vi "Autonomous Independent.vi"() -> ()   [LabVIEW 2012]
doc: "This VI is called when autonomous begins, and will automatically be terminated when autonomous ends. You can carry out timed or sensor driven robot movement independently without needing to return to the caller."
uses:
  <vilib>/Rock Robotics/WPI/RobotDrive/WPI_RobotDriveArcadeDrive_Standard(NoSaturation).vi
  Robot Global Data.vi
  <vilib>/Rock Robotics/WPI/Solenoid/WPI_SolenoidSetEnum.vi
  <vilib>/Rock Robotics/WPI/Solenoid/WPI_SolenoidValue.ctl
  <vilib>/Rock Robotics/WPI/CAN/Jaguar/SubVIs/WPI_CANJaguar_ControlMode.ctl
  <vilib>/Rock Robotics/WPI/CAN/Jaguar/SubVIs/WPI_CANJaguar_PositionReference.ctl
panel:
  out "Current Movement, for debugging":T1 {"Y Joystick Value" scale=1.0..-1.0; "X Joystick Value" scale=-1.0..1.0}
  in  "Array of robot movements":T2(array[cluster]) {"Y Joystick Value" scale=1.0..-1.0; "X Joystick Value" scale=-1.0..1.0}
  # "Be sure to right-click and choose Data Operations>>Make Current Value default if you want to save the array values with the VI"
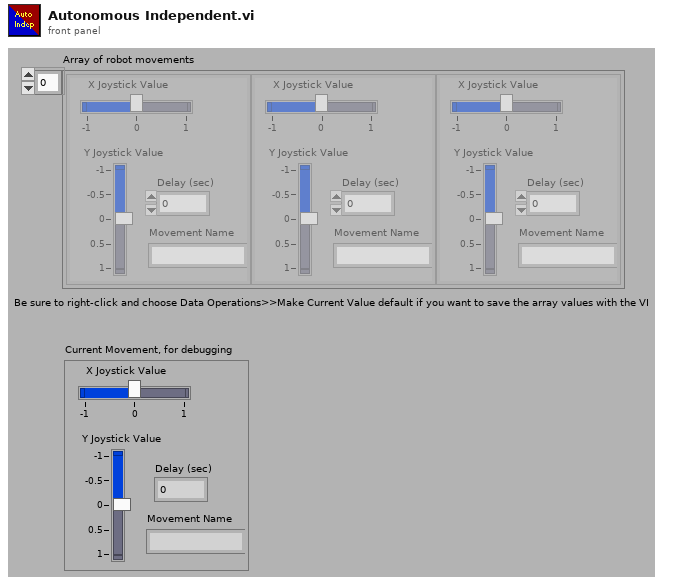
[diagram p1: front panel]
types:
  T1 = cluster{"X Joystick Value":dbl, "Y Joystick Value":dbl, "Delay (sec)":dbl, "Movement Name":string}
  T2 = cluster{"X Joystick Value":dbl, "Y Joystick Value":dbl, "Delay (sec)":dbl, "Movement Name":string}[]
  T3 = typedef "WPI_JoystickDevRef.ctl" = cluster{"Device":T4}
  T4 = typedef "WPI_JoystickDeviceEnum.ctl" = enum16{"USB 1", "USB 2", "USB 3", "USB 4", "Kinect 1", "Kinect 2"}
  T5 = cluster{"axis 1 (x)":dbl, "axis 2 (y)":dbl, "axis 3 (throttle)":dbl, "axis 4":dbl, "axis 5":dbl, "axis 6":dbl}
  T6 = typedef "WPI_SolenoidValue.ctl" = enum16{"Off", "On", "Forward", "Reverse"}
  T7 = typedef "WPI_CANJaguar_ControlMode.ctl" = enum8{"Percent VBus", "Current", "Speed", "Position", "Voltage"}
  T8 = typedef "WPI_SolenoidDevRef.ctl" = cluster{"DevStatus":errorcluster, "Solenoid Module":T9, "Forward Solenoid Channel":T10, "Reverse Solenoid Channel":T10}
  T9 = typedef "FPGA_TypedefSolenoidModule.ctl" = enum16{"Solenoid Module 1", "Solenoid Module 2"}
  T10 = typedef "WPI_SolenoidChannel.ctl" = enum8{"Solenoid 1", "Solenoid 2", "Solenoid 3", "Solenoid 4", "Solenoid 5", "Solenoid 6", "Solenoid 7", "Solenoid 8", "Invalid"}
  T11 = typedef "WPI_MotorControlDeviceRef.ctl" = cluster{"DeviceStatus":errorcluster, "Type":enum16{"PWM", "CAN"}, "PWM":cluster{"Digital Module":T12, "PWM Channel":T13, "DeadBand":T14}, "CAN":cluster{"Device Number":u8, "Control Mode":T7, "Semaphore":T15, "Max Vout":dbl}, "Invert":bool, "TransformRef":T16, "InvTransformRef":T16}
  T12 = typedef "FPGA_TypedefDigitalModule.ctl" = enum16{"Digital Module 1", "Digital Module 2"}
  T13 = typedef "FPGA_DIOPWMChannel.ctl" = enum8{"PWM 1", "PWM 2", "PWM 3", "PWM 4", "PWM 5", "PWM 6", "PWM 7", "PWM 8", "PWM 9", "PWM 10", "Invalid"}
  T14 = typedef "WPI_PWMDeadband.ctl" = cluster{"Name":string, "maxPositivePwm":i32, "minPositivePwm":i32, "centerPwm":i32, "maxNegativePwm":i32, "minNegativePwm":i32, "angularRange":u16}
  T15 = typedef "Semaphore RefNum" = refnum<k1>
  T16 = typedef "WPI_PWMTransform_ConPane.ctl" = refnum<vi>
  T17 = typedef "WPI_CANJaguar_PositionReference.ctl" = u8
  T18 = typedef "WPI_RobotDriveDevRef.ctl" = cluster{"DevStatus":errorcluster, "Motors[]":T11[], "Square Inputs":bool, "Max Output":dbl, "Isochronous":bool}
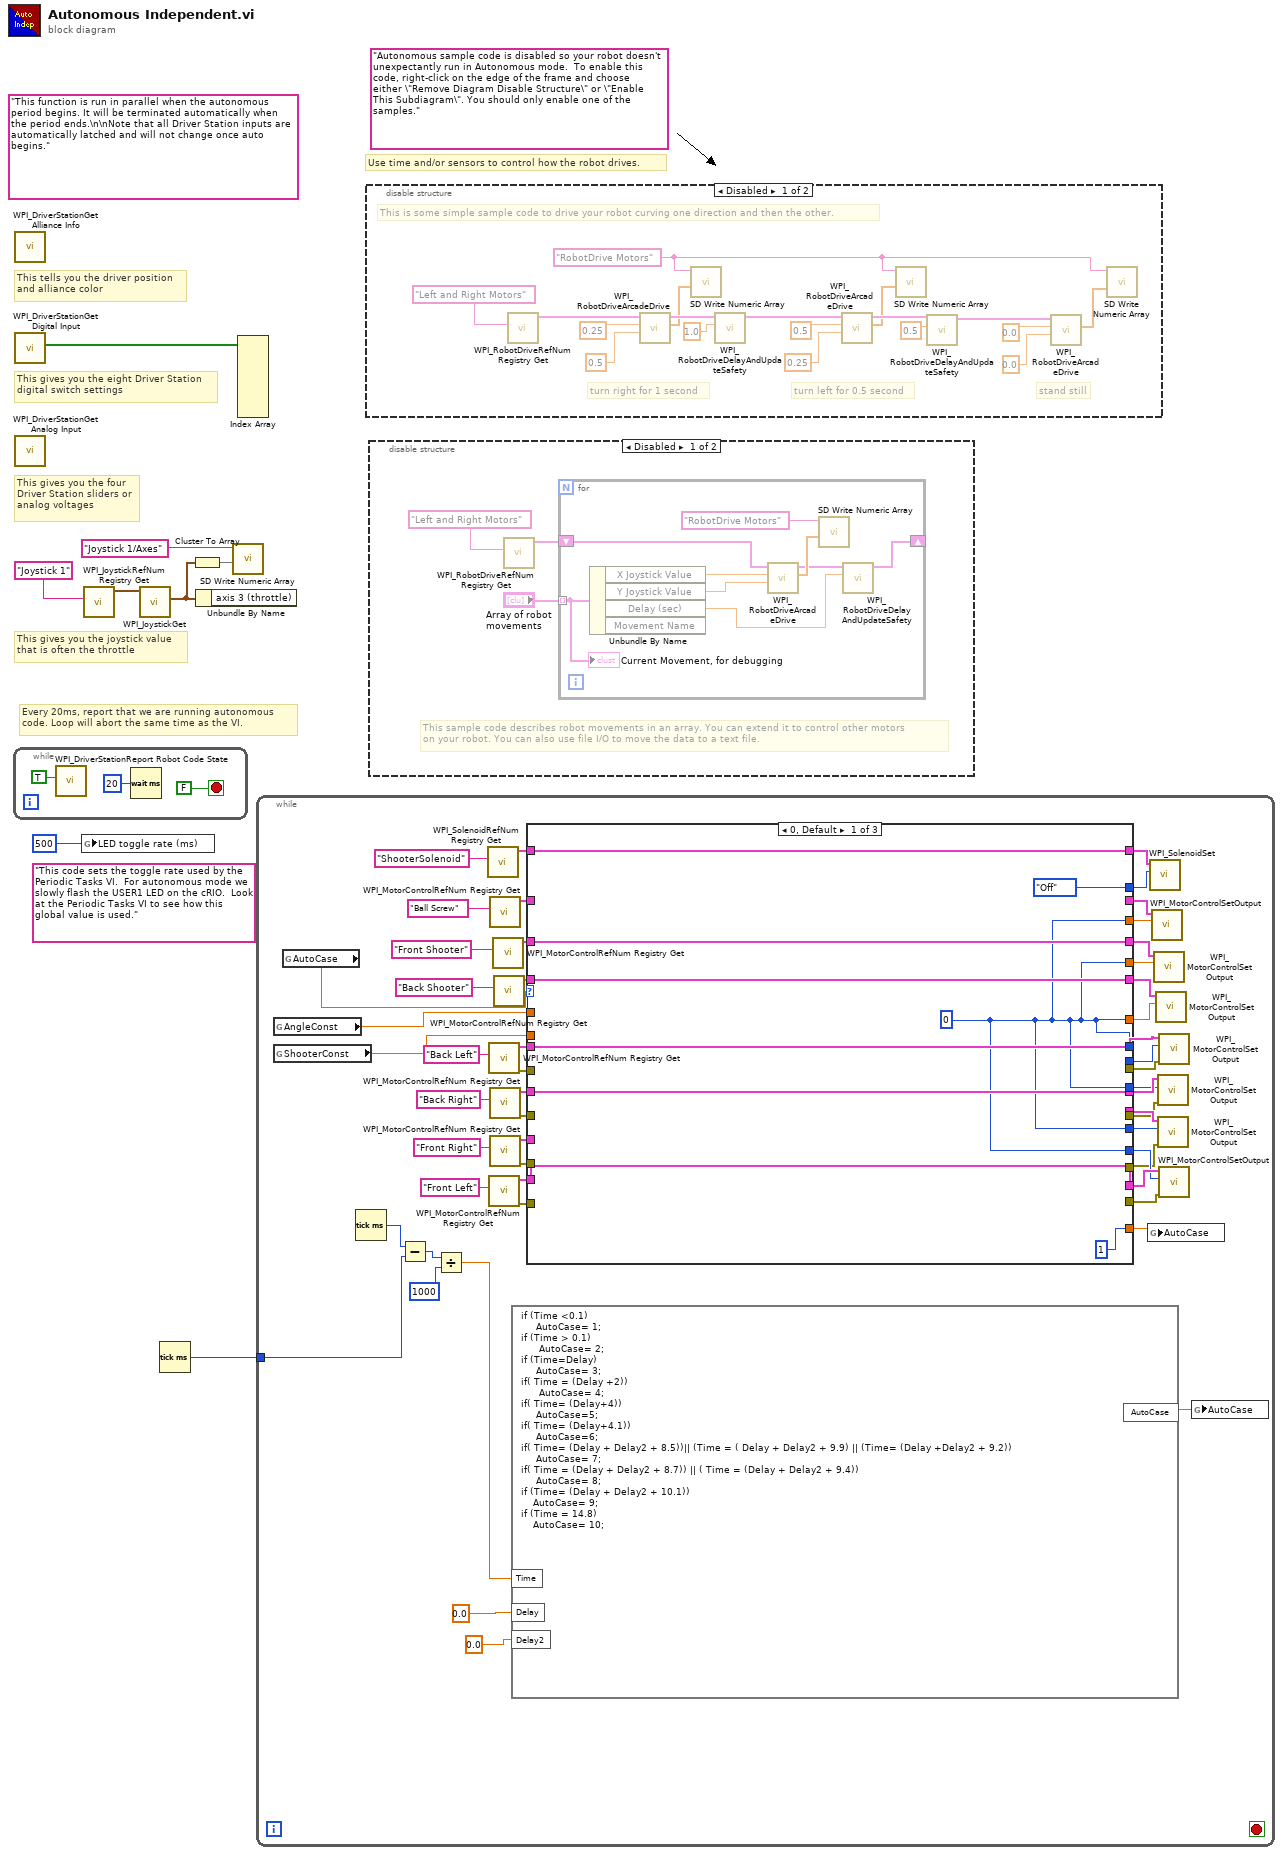
[diagram p0: block diagram]
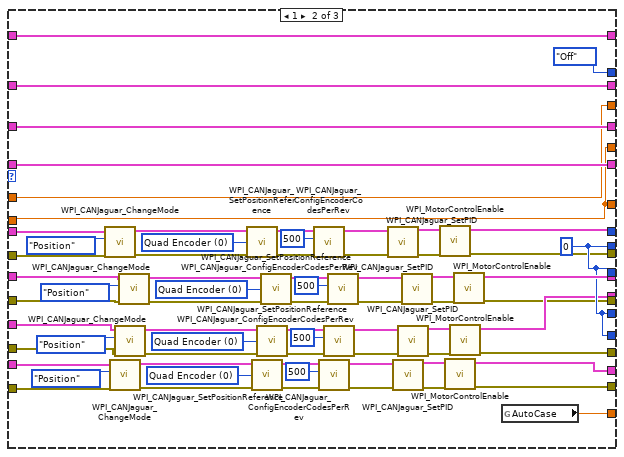
[diagram p2: hidden frame]
diagram:
  (unwired) "This code sets the toggle rate used by the Periodic Tasks VI.  For autonomous mode we slowly flash the USER1 LED on the cRIO.  Look at the Periodic Tasks VI to see how this global value is used."
  (unwired) "Autonomous sample code is disabled so your robot doesn't unexpectantly run in Autonomous mode.  To enable this code, right-click on the edge of the frame and choose either \"Remove Diagram Disable Structure\" or \"Enable This Subdiagram\". You should only enable one of the samples."
  (unwired) "This function is run in parallel when the autonomous period begins. It will be terminated automatically when the period ends.\n\nNote that all Driver Station inputs are automatically latched and will not change once auto begins."
  # "Every 20ms, report that we are running autonomous\ncode. Loop will abort the same time as the VI."
  # "This gives you the joystick value\nthat is often the throttle"
  # "Use time and/or sensors to control how the robot drives."
  # "This tells you the driver position\nand alliance color"
  # "This gives you the eight Driver Station\ndigital switch settings"
  # "This gives you the four\nDriver Station sliders or\nanalog voltages"
  n1 = while {
    stop <- FALSE stop-if-true
    n2 = call <vilib>:"WPI_DriverStationReport Robot Code State.vi"("Autonomous"=TRUE) -> ()  [unwired: 10 in, 1 out]
    n3 = Wait (ms)(milliseconds to wait=u32 20) -> ()  [unwired: 1 out]
  }
  n4 = call <vilib>:"WPI_DriverStationGet Alliance Info.vi"() -> ()  [unwired: 12 out]
  n5 = call <vilib>:"WPI_DriverStationGet Digital Input.vi"() -> ("Driver Station Digital Input (1-8)"=w8:bool[])  [unwired: 11 out]
  n6 = call <vilib>:"WPI_DriverStationGet Analog Input.vi"() -> ()  [unwired: 12 out]
  n7 = global write "Robot Global Data.vi" "LED toggle rate (ms)"(u32 500 ("LED ms toggle rate")) -> ()
  n8 = call <vilib>:"WPI_JoystickRefNum Registry Get.vi"("refnum name"="Joystick 1") -> ("JoystickDevRef"=w6:T3)  [unwired: 1 in, 9 out]
  n9 = call <vilib>:"WPI_JoystickGet.vi"("JoystickDevRef"=w6) -> ("Axes"=w3:T5)  [unwired: 1 in, 5 out]
  n10 = Tick Count (ms)() -> (millisecond timer value=w1:u32)
  n11 = Cluster To Array(cluster=w3) -> (array=w4:dbl[])
  n12 = Unbundle By Name(w3) -> ()  [unwired: 1 out]
  n13 = call <vilib>:"SD Write Numeric Array.vi"("Numeric Array"=w4, "Name"="Joystick 1/Axes") -> ()  [unwired: 8 in, 2 out]
  n14 = Index Array(array=w8) -> ()  [unwired: 8 in, 8 out]
  n15 = while {
    tunnel: w1 -> [w52]
    stop <- _ stop-if-true
    n16 = global read "Robot Global Data.vi" "AngleConst"() -> (w13:dbl)
    n17 = global read "Robot Global Data.vi" "ShooterConst"() -> (w12:dbl)
    n18 = global read "Robot Global Data.vi" "AutoCase"() -> (w54:dbl)
    n19 = Tick Count (ms)() -> (millisecond timer value=w53:u32)
    n20 = Subtract(x=w53, y=w52) -> (x-y=w51:u32)
    n21 = Divide(x=w51, y=u32 1000) -> (x/y=w49:dbl)
    n22 = call <vilib>:"WPI_SolenoidRefNum Registry Get.vi"("refnum name"="ShooterSolenoid") -> ("SolenoidDevRef"=w55:T8)  [unwired: 9 in, 1 out]
    n23 = call <vilib>:"WPI_MotorControlRefNum Registry Get.vi"("refnum name"="Back Left") -> ("error out"=w25:errorcluster, "MotorControlDevRef"=w37:T11)  [unwired: 9 in]
    n24 = call <vilib>:"WPI_MotorControlRefNum Registry Get.vi"("refnum name"="Front Left") -> ("error out"=w15:errorcluster, "MotorControlDevRef"=w33:T11)  [unwired: 9 in]
    n25 = call <vilib>:"WPI_MotorControlRefNum Registry Get.vi"("refnum name"="Ball Screw") -> ("MotorControlDevRef"=w26:T11)  [unwired: 9 in, 1 out]
    n26 = call <vilib>:"WPI_MotorControlRefNum Registry Get.vi"("refnum name"="Back Right") -> ("error out"=w23:errorcluster, "MotorControlDevRef"=w35:T11)  [unwired: 9 in]
    n27 = call <vilib>:"WPI_MotorControlRefNum Registry Get.vi"("refnum name"="Front Right") -> ("error out"=w19:errorcluster, "MotorControlDevRef"=w21:T11)  [unwired: 9 in]
    n28 = call <vilib>:"WPI_MotorControlRefNum Registry Get.vi"("refnum name"="Front Shooter") -> ("MotorControlDevRef"=w41:T11)  [unwired: 9 in, 1 out]
    n29 = call <vilib>:"WPI_MotorControlRefNum Registry Get.vi"("refnum name"="Back Shooter") -> ("MotorControlDevRef"=w39:T11)  [unwired: 9 in, 1 out]
    n30 = formula code="if (Time <0.1)\n     AutoCase= 1;\nif (Time > 0.1)\n      AutoCase= 2;\nif (Time=Delay)\n     AutoCase= 3;\nif( Time = (Delay +2))\n      AutoCase= 4;\nif( Time= (Delay+4))\n     AutoCase=5;\nif( Time= (Delay+4.1))\n     AutoCase=6;\nif( Time= (Delay + Delay2 + 8.5))|| (Time = ( Delay + Delay2 + 9.9) || (Time= (Delay +Delay2 + 9.2))\n     AutoCase= 7;\nif( Time = (Delay + Delay2 + 8.7)) || ( Time = (Delay + Delay2 + 9.4))\n     AutoCase= 8;\nif (Time= (Delay + Delay2 + 10.1))\n    AutoCase= 9;\nif (Time = 14.8)\n    AutoCase= 10;"("Time"=w49, "Delay"=0.0 ("input variable"), "Delay2"=0.0 ("input variable")) -> ("AutoCase"=w48:dbl)
    n31 = case shown="0, Default" w54 {
      tunnel: w55 -> [w70 w139 _]
      tunnel: [1 w141 _] -> w45
      tunnel: [WPI_SolenoidValue."Off" ("Value") WPI_SolenoidValue."Off" ("Value") _] -> w44
      tunnel: [w70 w139 _] -> w43
      tunnel: [_ w128 _] -> w42
      tunnel: [w69 w76 _] -> w40
      tunnel: w41 -> [w69 w76 _]
      tunnel: [w68 w75 _] -> w38
      tunnel: w39 -> [w68 w75 _]
      tunnel: [w67 w124 _] -> w36
      tunnel: w37 -> [w67 w129 _]
      tunnel: [w66 w110 _] -> w34
      tunnel: w35 -> [w66 w112 _]
      tunnel: [w65 w78 _] -> w32
      tunnel: w33 -> [w65 w80 _]
      tunnel: [w64 w73 _] -> w30
      tunnel: [w64 w74 _] -> w31
      tunnel: [w64 w73 _] -> w29
      tunnel: [w64 _ _] -> _
      tunnel: [w64 w109 _] -> w28
      tunnel: [w64 w109 _] -> w27
      tunnel: w26 -> [_ w128 _]
      tunnel: w25 -> [_ w125 _]
      tunnel: [_ w109 _] -> w24
      tunnel: w23 -> [_ w111 _]
      tunnel: [w64 w109 _] -> w22
      tunnel: w21 -> [_ w97 _]
      tunnel: [_ w96 _] -> w20
      tunnel: w19 -> [_ w95 _]
      tunnel: [_ w94 _] -> w18
      tunnel: [_ w93 _] -> w17
      tunnel: [_ w92 _] -> w16
      tunnel: w15 -> [_ w79 _]
      tunnel: [_ w77 _] -> w14
      tunnel: w13 -> [_ w74 _]
      tunnel: w12 -> [_ w73 _]
      frame 0, Default {
        w64 = 0
      }
      frame 1 {
        w88 = T17 0 items=["Quad Encoder"=0, "Potentiometer"=1, "None"=255] ("Position Reference")
        w105 = T17 0 items=["Quad Encoder"=0, "Potentiometer"=1, "None"=255] ("Position Reference")
        w120 = T17 0 items=["Quad Encoder"=0, "Potentiometer"=1, "None"=255] ("Position Reference")
        w109 = 0
        w135 = T17 0 items=["Quad Encoder"=0, "Potentiometer"=1, "None"=255] ("Position Reference")
        n32 = call <vilib>:"WPI_CANJaguar_ChangeMode.vi"("error in (no error)"=w125, "Control Mode"=WPI_CANJaguar_ControlMode."Position", "CAN Jaguar Ref"=w129) -> ("error out"=w137:errorcluster, "CAN Jaguar Ref Out"=w136:T11)  [unwired: 7 in]
        n33 = call <vilib>:"WPI_CANJaguar_ChangeMode.vi"("error in (no error)"=w79, "Control Mode"=WPI_CANJaguar_ControlMode."Position", "CAN Jaguar Ref"=w80) -> ("error out"=w90:errorcluster, "CAN Jaguar Ref Out"=w89:T11)  [unwired: 7 in]
        n34 = call <vilib>:"WPI_CANJaguar_ChangeMode.vi"("error in (no error)"=w95, "Control Mode"=WPI_CANJaguar_ControlMode."Position", "CAN Jaguar Ref"=w97) -> ("error out"=w107:errorcluster, "CAN Jaguar Ref Out"=w106:T11)  [unwired: 7 in]
        n35 = call <vilib>:"WPI_CANJaguar_ChangeMode.vi"("error in (no error)"=w111, "Control Mode"=WPI_CANJaguar_ControlMode."Position", "CAN Jaguar Ref"=w112) -> ("error out"=w122:errorcluster, "CAN Jaguar Ref Out"=w121:T11)  [unwired: 7 in]
        n36 = call <vilib>:"WPI_CANJaguar_SetPositionReference.vi"("error in (no error)"=w137, "Position Reference"=w135, "CAN Jaguar Ref"=w136) -> ("error out"=w132:errorcluster, "CAN Jaguar Ref Out"=w134:T11)  [unwired: 7 in]
        n37 = call <vilib>:"WPI_CANJaguar_SetPositionReference.vi"("error in (no error)"=w90, "Position Reference"=w88, "CAN Jaguar Ref"=w89) -> ("error out"=w85:errorcluster, "CAN Jaguar Ref Out"=w87:T11)  [unwired: 7 in]
        n38 = call <vilib>:"WPI_CANJaguar_SetPositionReference.vi"("error in (no error)"=w107, "Position Reference"=w105, "CAN Jaguar Ref"=w106) -> ("error out"=w102:errorcluster, "CAN Jaguar Ref Out"=w104:T11)  [unwired: 7 in]
        n39 = call <vilib>:"WPI_CANJaguar_SetPositionReference.vi"("error in (no error)"=w122, "Position Reference"=w120, "CAN Jaguar Ref"=w121) -> ("error out"=w117:errorcluster, "CAN Jaguar Ref Out"=w119:T11)  [unwired: 7 in]
        n40 = call <vilib>:"WPI_CANJaguar_ConfigEncoderCodesPerRev.vi"("error in (no error)"=w132, "Encoder Codes Per Rev"=u16 500, "CAN Jaguar Ref"=w134) -> ("error out"=w130:errorcluster, "CAN Jaguar Ref Out"=w131:T11)  [unwired: 7 in]
        n41 = call <vilib>:"WPI_CANJaguar_ConfigEncoderCodesPerRev.vi"("error in (no error)"=w85, "Encoder Codes Per Rev"=u16 500, "CAN Jaguar Ref"=w87) -> ("error out"=w83:errorcluster, "CAN Jaguar Ref Out"=w84:T11)  [unwired: 7 in]
        n42 = call <vilib>:"WPI_CANJaguar_ConfigEncoderCodesPerRev.vi"("error in (no error)"=w102, "Encoder Codes Per Rev"=u16 500, "CAN Jaguar Ref"=w104) -> ("error out"=w100:errorcluster, "CAN Jaguar Ref Out"=w101:T11)  [unwired: 7 in]
        n43 = call <vilib>:"WPI_CANJaguar_ConfigEncoderCodesPerRev.vi"("error in (no error)"=w117, "Encoder Codes Per Rev"=u16 500, "CAN Jaguar Ref"=w119) -> ("error out"=w115:errorcluster, "CAN Jaguar Ref Out"=w116:T11)  [unwired: 7 in]
        n44 = call <vilib>:"WPI_CANJaguar_SetPID.vi"("CAN Jaguar Ref"=w131, "error in (no error)"=w130) -> ("CAN Jaguar Ref Out"=w126:T11, "error out"=w127:errorcluster)  [unwired: 12 in]
        n45 = call <vilib>:"WPI_CANJaguar_SetPID.vi"("CAN Jaguar Ref"=w84, "error in (no error)"=w83) -> ("CAN Jaguar Ref Out"=w81:T11, "error out"=w82:errorcluster)  [unwired: 12 in]
        n46 = call <vilib>:"WPI_CANJaguar_SetPID.vi"("CAN Jaguar Ref"=w101, "error in (no error)"=w100) -> ("CAN Jaguar Ref Out"=w98:T11, "error out"=w99:errorcluster)  [unwired: 12 in]
        n47 = call <vilib>:"WPI_CANJaguar_SetPID.vi"("CAN Jaguar Ref"=w116, "error in (no error)"=w115) -> ("CAN Jaguar Ref Out"=w113:T11, "error out"=w114:errorcluster)  [unwired: 12 in]
        n48 = call <vilib>:"WPI_MotorControlEnable.vi"("error in (no error)"=w127, "CAN Jaguar Ref"=w126) -> ("error out"=w94:errorcluster, "CAN Jaguar Ref Out"=w124:T11)  [unwired: 8 in]
        n49 = call <vilib>:"WPI_MotorControlEnable.vi"("error in (no error)"=w82, "CAN Jaguar Ref"=w81) -> ("error out"=w77:errorcluster, "CAN Jaguar Ref Out"=w78:T11)  [unwired: 8 in]
        n50 = call <vilib>:"WPI_MotorControlEnable.vi"("error in (no error)"=w99, "CAN Jaguar Ref"=w98) -> ("error out"=w92:errorcluster, "CAN Jaguar Ref Out"=w96:T11)  [unwired: 8 in]
        n51 = call <vilib>:"WPI_MotorControlEnable.vi"("error in (no error)"=w114, "CAN Jaguar Ref"=w113) -> ("error out"=w93:errorcluster, "CAN Jaguar Ref Out"=w110:T11)  [unwired: 8 in]
        n52 = global read "Robot Global Data.vi" "AutoCase"() -> (w141:dbl)
      }
      frame 2 {
      }
    }
    n53 = global write "Robot Global Data.vi" "AutoCase"(w45) -> ()
    n54 = call-poly <vilib>:"WPI_SolenoidSet.vi"("Value"=w44, "SolenoidDevRef"=w43) -> ()  [unwired: 8 in, 2 out]
    n55 = call <vilib>:"WPI_MotorControlSetOutput.vi"("Output"=w31, "MotorControlDevRef"=w42) -> ()  [unwired: 7 in, 3 out]
    n56 = call <vilib>:"WPI_MotorControlSetOutput.vi"("Output"=w29, "MotorControlDevRef"=w40) -> ()  [unwired: 7 in, 3 out]
    n57 = call <vilib>:"WPI_MotorControlSetOutput.vi"("Output"=w30, "MotorControlDevRef"=w38) -> ()  [unwired: 7 in, 3 out]
    n58 = call <vilib>:"WPI_MotorControlSetOutput.vi"("error in (no error)"=w17, "Output"=w28, "MotorControlDevRef"=w34) -> ()  [unwired: 6 in, 3 out]
    n59 = call <vilib>:"WPI_MotorControlSetOutput.vi"("error in (no error)"=w16, "Output"=w27, "MotorControlDevRef"=w20) -> ()  [unwired: 6 in, 3 out]
    n60 = call <vilib>:"WPI_MotorControlSetOutput.vi"("error in (no error)"=w18, "Output"=w24, "MotorControlDevRef"=w36) -> ()  [unwired: 6 in, 3 out]
    n61 = call <vilib>:"WPI_MotorControlSetOutput.vi"("error in (no error)"=w14, "Output"=w22, "MotorControlDevRef"=w32) -> ()  [unwired: 6 in, 3 out]
    n62 = global write "Robot Global Data.vi" "AutoCase"(w48) -> ()
  }
  n63 = disable-structure shown="Disabled" {
    frame Disabled {
      w142 = "RobotDrive Motors" ("Name")
      # "This is some simple sample code to drive your robot curving one direction and then the other."
      # "stand still"
      # "turn left for 0.5 second"
      # "turn right for 1 second"
      n64 = call <vilib>:"WPI_RobotDriveRefNum Registry Get.vi"("refnum name"="Left and Right Motors") -> ("RobotDriveDevRef"=w146:T18)  [unwired: 1 in, 9 out]
      n65 = call-poly <vilib>:"WPI_RobotDriveArcadeDrive.vi"("Y axis value"=0.5 ("X axis value"), "X axis value"=0.25, "RobotDriveDevRef"=w146) -> ("Motor Values"=w145:dbl[], "RobotDriveDevRef"=w153:T18)  [unwired: 1 in, 6 out]
      n66 = call <vilib>:"SD Write Numeric Array.vi"("Numeric Array"=w145, "Name"=w142) -> ()  [unwired: 8 in, 2 out]
      n67 = call <vilib>:"WPI_RobotDriveDelayAndUpdateSafety.vi"("Delay (s)"=1.0, "RobotDriveDevRef"=w153) -> ("RobotDriveDevRef 2"=w152:T18)  [unwired: 8 in, 1 out]
      n68 = call-poly <vilib>:"WPI_RobotDriveArcadeDrive.vi"("Y axis value"=0.25 ("X axis value"), "X axis value"=0.5, "RobotDriveDevRef"=w152) -> ("Motor Values"=w144:dbl[], "RobotDriveDevRef"=w151:T18)  [unwired: 1 in, 6 out]
      n69 = call <vilib>:"SD Write Numeric Array.vi"("Numeric Array"=w144, "Name"=w142) -> ()  [unwired: 8 in, 2 out]
      n70 = call <vilib>:"WPI_RobotDriveDelayAndUpdateSafety.vi"("Delay (s)"=0.5, "RobotDriveDevRef"=w151) -> ("RobotDriveDevRef 2"=w150:T18)  [unwired: 8 in, 1 out]
      n71 = call-poly <vilib>:"WPI_RobotDriveArcadeDrive.vi"("Y axis value"=0.0 ("X axis value"), "X axis value"=0.0, "RobotDriveDevRef"=w150) -> ("Motor Values"=w143:dbl[])  [unwired: 1 in, 7 out]
      n72 = call <vilib>:"SD Write Numeric Array.vi"("Numeric Array"=w143, "Name"=w142) -> ()  [unwired: 8 in, 2 out]
    }
    frame Enabled {
    }
  }
  n73 = disable-structure shown="Disabled" {
    frame Disabled {
      # "This sample code describes robot movements in an array. You can extend it to control other motors\non your robot. You can also use file I/O to move the data to a text file."
      n74 = call <vilib>:"WPI_RobotDriveRefNum Registry Get.vi"("refnum name"="Left and Right Motors") -> ("RobotDriveDevRef"=w161:T18)  [unwired: 1 in, 9 out]
      n75 = for {
        shift-right: [w167] -> _
        shift-left: w161 -> [w168]
        tunnel: "Array of robot movements" -> [w163] mode=indexing
        n76 = Unbundle By Name(w163) -> ("X Joystick Value"=w166:dbl, "Y Joystick Value"=w165:dbl, "Delay (sec)"=w164:dbl)  [unwired: 1 out]
        n77 = call-poly <vilib>:"WPI_RobotDriveArcadeDrive.vi"("Y axis value"=w165, "X axis value"=w166, "RobotDriveDevRef"=w168) -> ("Motor Values"=w170:dbl[], "RobotDriveDevRef"=w169:T18)  [unwired: 1 in, 6 out]
        n78 = call <vilib>:"SD Write Numeric Array.vi"("Numeric Array"=w170, "Name"="RobotDrive Motors") -> ()  [unwired: 8 in, 2 out]
        n79 = call <vilib>:"WPI_RobotDriveDelayAndUpdateSafety.vi"("Delay (s)"=w164, "RobotDriveDevRef"=w169) -> ("RobotDriveDevRef 2"=w167:T18)  [unwired: 8 in, 1 out]
        "Current Movement, for debugging" <- w163
      }
    }
    frame Enabled {
    }
  }
